vi "FilterClusterArray.vi"(1 "Ys IN":dbl[][](array[numeric]), 2 "X IN":dbl[](array[numeric])) -> (0 "OUT":dbl[][](array[numeric]))   [LabVIEW 2023]
uses:
  eb81d46f-71f3-0a4c-b475-802b59b9bc5c.vi
  <vilib>/Array/Sort 2D Array - Pop Stack.vi
  <vilib>/Array/Sort 2D Array - Push Stack.vi
  eb81d46f-71f3-0a4c-b475-802b59b9bc5c.vi/269d4b3b-47f5-49e3-8884-44851e4dd9d5.vi
  eb81d46f-71f3-0a4c-b475-802b59b9bc5c.vi/6d99389c-673d-4efb-bf33-19b32bcf4cf8.vi
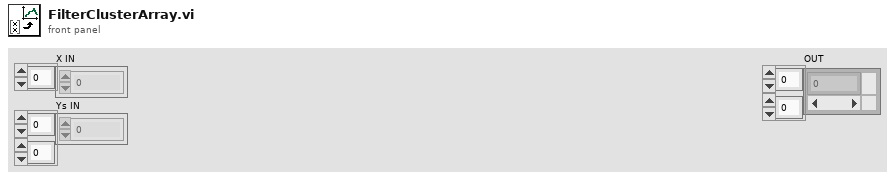
[diagram p1: front panel]
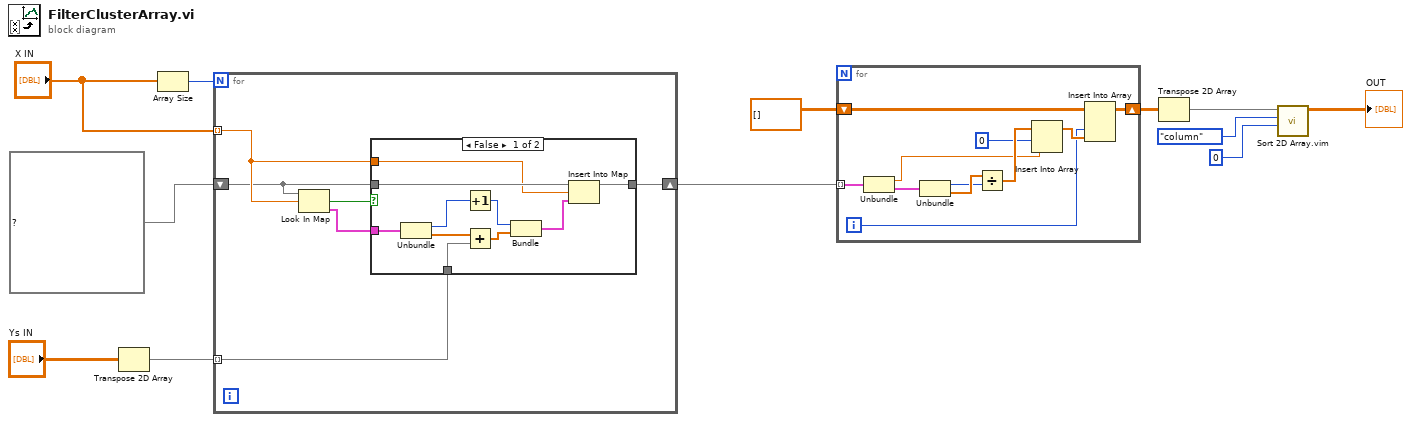
[diagram p0: block diagram]
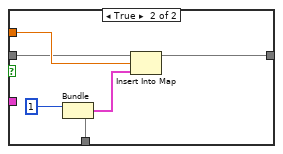
[diagram p2: hidden frame]
diagram:
  n1 = Transpose 2D Array(2D array="Ys IN") -> (transposed array=w10:dbl[][])
  n2 = Array Size(array="X IN") -> (size(s)=w12:i32)
  n3 = for {
    N: w12 -> [_]
    tunnel: "X IN" -> [w17] mode=indexing
    tunnel: w10 -> [w16] mode=indexing
    shift-right: [w14] -> w8
    shift-left: map{dbl, cluster{"Count":i32, "Ys":dbl[]}} {} ("map") -> [w13]
    n4 = Look In Map(map=w13, key=w17) -> (key not found?=w18:bool, value=w15:cluster{i32, dbl[]})  [unwired: 1 in]
    n5 = case shown="False" w18 {
      tunnel: w17 -> [w21 w34]
      tunnel: w13 -> [w22 w33]
      tunnel: w16 -> [w25 w31]
      tunnel: [w19 w29] -> w14
      tunnel: w15 -> [w28 _]
      frame False {
        n6 = Unbundle(w28) -> (w27:i32, w26:dbl[])
        n7 = Increment(x=w27) -> (x+1=w24:i32)
        n8 = Add(x=w26, y=w25) -> (x+y=w23:dbl[])
        n9 = Bundle(w24, w23) -> (w20:cluster{i32, dbl[]})  [unwired: 1 in]
        n10 = Insert Into Map(map in=w22, key=w21, value=w20) -> (map out=w19:map{dbl, cluster{"Count":i32, "Ys":dbl[]}})  [unwired: 2 out]
      }
      frame True {
        n11 = Bundle(1, w31) -> (w30:cluster{i32, dbl[]})  [unwired: 1 in]
        n12 = Insert Into Map(map in=w33, key=w34, value=w30) -> (map out=w29:map{dbl, cluster{"Count":i32, "Ys":dbl[]}})  [unwired: 2 out]
      }
    }
  }
  n13 = for {
    tunnel: w8 -> [w45] mode=indexing
    shift-right: [w36] -> w6
    shift-left: dbl[][] [] ("2D array") -> [w37]
    i -> [w35]
    n14 = Unbundle(w45) -> (w40:dbl, w44:cluster{"Count":i32, "Ys":dbl[]})
    n15 = Unbundle(w44) -> ("Count"=w42:i32, "Ys"=w43:dbl[])
    n16 = Divide(x=w43, y=w42) -> (x/y=w41:dbl[])
    n17 = Insert Into Array(array=w41, index=0, new element=w40) -> (w38:dbl[])
    n18 = Insert Into Array(array=w37, index (col)=w35, new element=w38) -> (w36:dbl[][])  [unwired: 1 in]
  }
  n19 = Transpose 2D Array(2D array=w6) -> (transposed array=w5:dbl[][])
  n20 = call "Sort 2D Array.vim"("index"=0, "dimension to index (column)"=enum16{"column", "row"}."column", "2D array"=w5) -> ("sorted 2D array"=→"OUT":dbl[][])  [unwired: 7 in, 1 out]
